vi "S2C_Access_DeleteTable.vi"(8 "Error In":errorcluster) -> (0 "Error Out":errorcluster, 3 "Canceled?":bool)   [LabVIEW 2015]
uses:
  S2C_Access_Select.ctl
  S2C_Access_Globals.vi
  <vilib>/addons/database/NI_Database_API.lvlib
panel:
  in  "Delete":bool
  in  "Tables":T1="<Select>" caption="Table Name"
  out "Init":bool
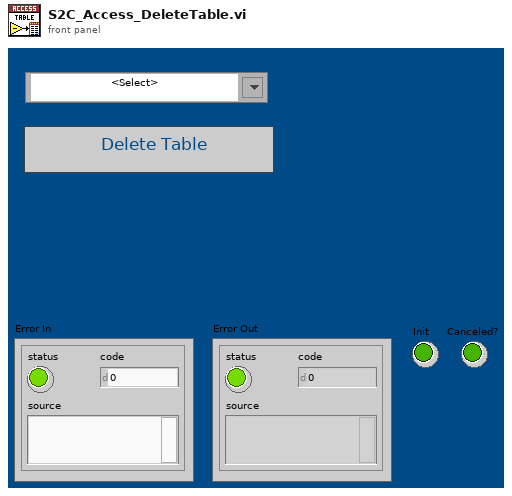
[diagram p1: front panel]
types:
  T1 = typedef "S2C_Access_Select.ctl" = string
  T2 = typedef "LVComboBoxStrsAndValuesArrayTypeDef.ctl" = cluster{"String":string, "Value":string}[]
  T3 = typedef "NI_Database_API.lvlib/Conn ObjectReference.ctl" = refnum<k1>
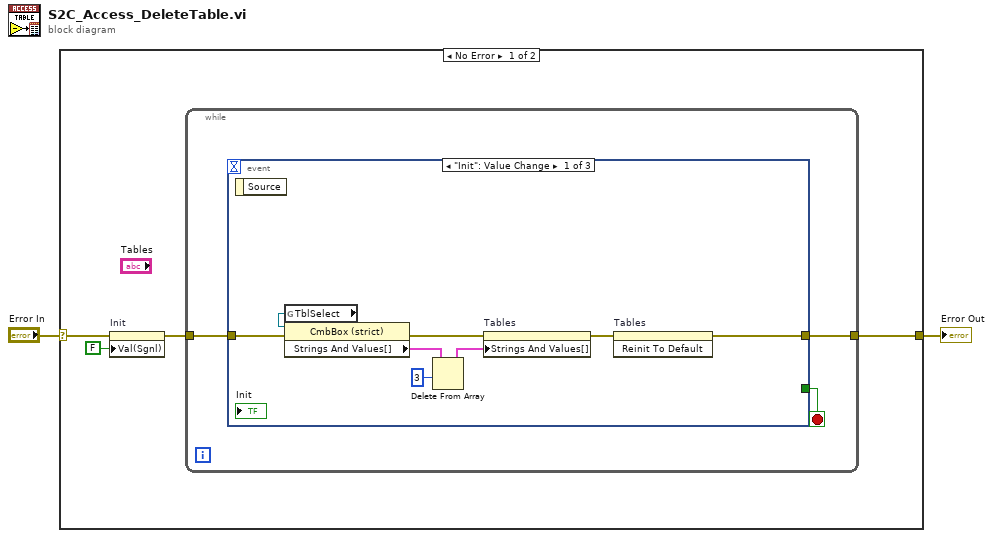
[diagram p0: block diagram]
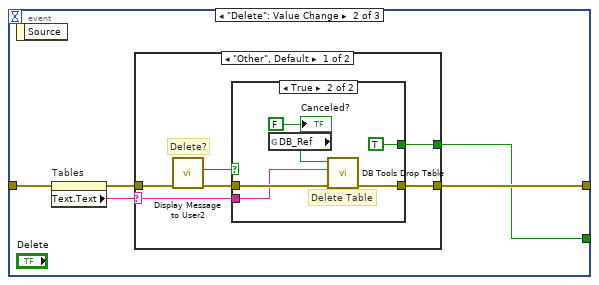
[diagram p2: hidden frame]
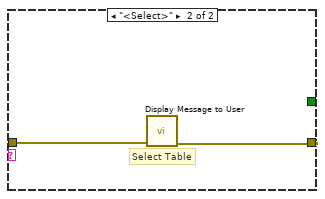
[diagram p4: hidden frame]
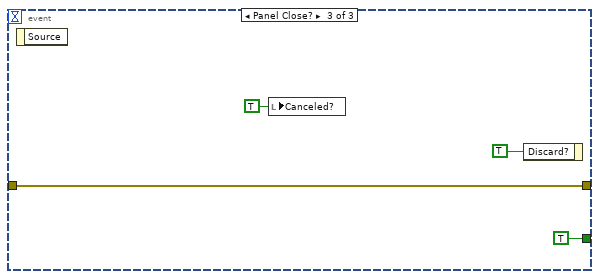
[diagram p5: hidden frame]
diagram:
  n1 = case shown="No Error" "Error In" {
    selector: "Error In" -> [w6 w42]
    tunnel: [w3 w42] -> w1
    frame No Error {
      n2 = property on="Init" class="Bool (strict)"(error in=w6, "Val(Sgnl)"=FALSE ("Value (Signaling)")) -> (error out=w5:errorcluster)  [unwired: 1 in, 1 out]
      n3 = while {
        tunnel: w5 -> [w9]
        tunnel: [w8] -> w3
        stop <- w7 stop-if-true
        n4 = event shown="[0] \"Init\": Value Change" {
          selector: _ -> [_ _ _]
          dyn-events: _ -> [_ _ _]
          timeout: _ -> [_ _ _]
          tunnel: w9 -> [w16 w21 w41]
          tunnel: [w13 w22 w41] -> w8
          tunnel: [_ w18 TRUE] -> w7
          event "Init": Value Change {
            n5 = event-data() -> ()  [unwired: 1 in, 1 out]
            n6 = global read "S2C_Access_Globals.vi" "TblSelect"() -> (w17:refnum<vi>)
            n7 = property class="CmbBox (strict)"(reference=w17, error in=w16) -> (error out=w15:errorcluster, "Strings And Values[]"=w12:T2)  [unwired: 1 out]
            n8 = Delete From Array(array=w12, length=3) -> (array with subset deleted=w11:T2)  [unwired: 1 in, 1 out]
            n9 = property on="Tables" class="CmbBox (strict)"(error in=w15, "Strings And Values[]"=w11) -> (error out=w14:errorcluster)  [unwired: 1 in, 1 out]
            n10 = invoke on="Tables" class="CmbBox (strict)" method="Reinit To Default"(error in=w14) -> (error out=w13:errorcluster)  [unwired: 2 in, 2 out]
          }
          event "Delete": Value Change {
            n11 = event-data() -> ()  [unwired: 1 in, 1 out]
            n12 = property on="Tables" class="CmbBox (strict)"(error in=w21) -> (error out=w20:errorcluster, "Text.Text"=w19:string)  [unwired: 1 in, 1 out]
            n13 = case shown="\"Other\", Default" w19 {
              selector: w19 -> [w24 _]
              tunnel: [w28 w36] -> w22
              tunnel: w20 -> [w27 w37]
              tunnel: [w23 _] -> w18
              frame "Other", Default {
                # "Delete?"
                n14 = call "Display Message to User2"("error in (no error)"=w27) -> ("error out"=w26:errorcluster, "Delete"=w25:bool)  [unwired: 9 in]
                n15 = case shown="True" w25 {
                  tunnel: w26 -> [w29 w33]
                  tunnel: [w29 w34] -> w28
                  tunnel: w24 -> [_ w32]
                  tunnel: [_ TRUE] -> w23
                  frame False {
                  }
                  frame True {
                    # "Delete Table"
                    n16 = global read "S2C_Access_Globals.vi" "DB_Ref"() -> (w35:T3)
                    n17 = call <vilib>:"DB Tools Drop Table.vi"("error in (no error)"=w33, "table"=w32, "connection reference"=w35) -> ("error out"=w34:errorcluster)  [unwired: 5 in, 1 out]
                    "Canceled?" <- FALSE ("Canceled?")
                  }
                }
              }
              frame "<Select>" {
                # "Select Table"
                n18 = call "Display Message to User"("error in (no error)"=w37) -> ("error out"=w36:errorcluster)  [unwired: 9 in, 1 out]
              }
            }
          }
          event Panel Close? {
            n19 = event-data() -> ()  [unwired: 1 in, 1 out]
            n20 = local write "Canceled?"(TRUE ("Canceled?")) -> ()
            n21 = event-data("Discard?"=TRUE) -> ()  [unwired: 1 in, 1 out]
          }
        }
      }
    }
    frame Error {
    }
  }
  "Error Out" <- w1
